vi "Parse HEARTBEAT.vi"(11 "Data":string) -> (3 "Heartbeat":T1 {"custom_mode" format="%x"})   [LabVIEW 2014]
uses:
  Controls/MAVLink Heartbeat.ctl
panel:
  out "Cutom Mode":u32
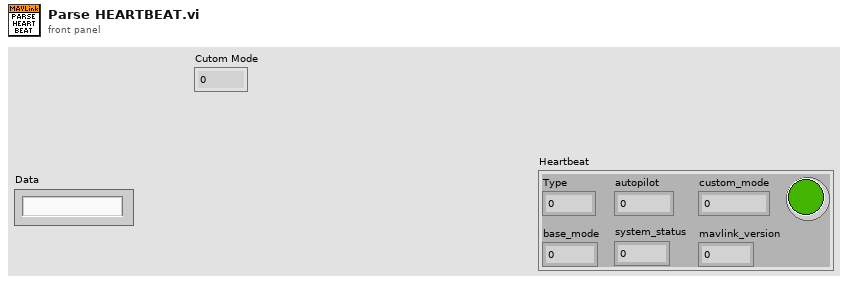
[diagram p1: front panel]
types:
  T1 = typedef "MAVLink Heartbeat.ctl" = cluster{"custom_mode":u32, "Type":u8, "autopilot":u8, "base_mode":u8, "system_status":u8, "mavlink_version":u8, "heartbeat":bool}
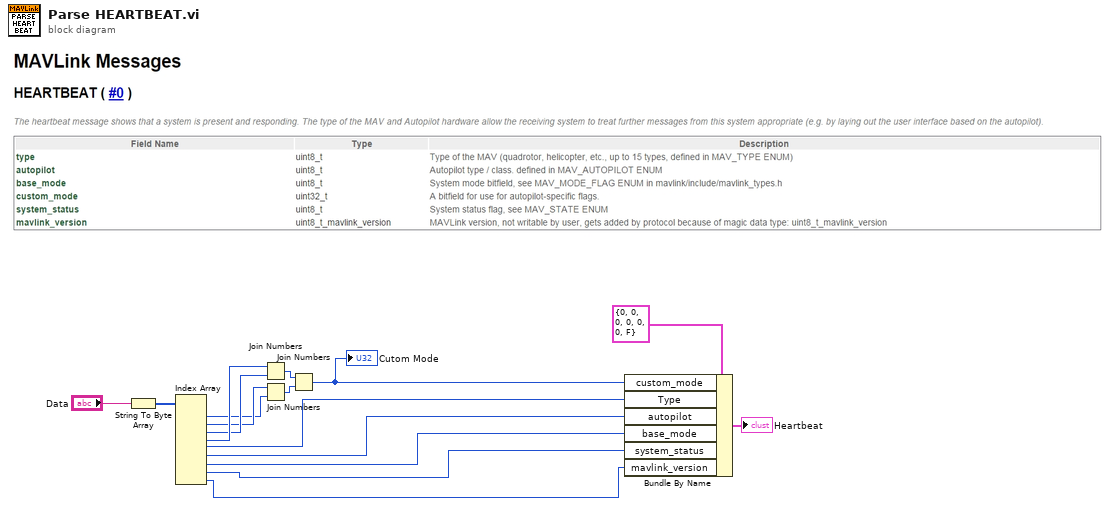
[diagram p0: block diagram]
diagram:
  n1 = String To Byte Array(string="Data") -> (unsigned byte array=w10:u8[])
  n2 = Index Array(array=w10) -> (element #1=w11:u8, element #2=w12:u8, element #3=w13:u8, element #4=w14:u8, element #5=w6:u8, element #6=w5:u8, element #7=w4:u8, element #8=w3:u8, element #9=w2:u8)  [unwired: 9 in]
  n3 = Join Numbers(hi=w14, lo=w13) -> ((hi.lo)=w16:u16)
  n4 = Join Numbers(hi=w12, lo=w11) -> ((hi.lo)=w15:u16)
  n5 = Join Numbers(hi=w16, lo=w15) -> ((hi.lo)=w7:u32)
  "Cutom Mode" <- w7
  n6 = Bundle By Name(cluster=T1 {"custom_mode"=0, "Type"=0, "autopilot"=0, "base_mode"=0, "system_status"=0, "mavlink_version"=0, "heartbeat"=FALSE} ("HeartBeat"), "custom_mode"=w7, "Type"=w6, "autopilot"=w5, "base_mode"=w4, "system_status"=w3, "mavlink_version"=w2) -> (→"Heartbeat":T1)
